vi "Set Channel by Name.vi"(8 "error in":errorcluster, 9 "Target":dbl, 10 "Channel Name":string, 11 "PRM in":refnum<class "PRM.lvclass">) -> (0 "error out":errorcluster, 3 "PRM out":refnum<class "PRM.lvclass">)   [LabVIEW 2019, in "PRM.lvlib" / "PRM.lvclass"]
uses:
  Library/PRM.lvclass
  C:/Users/Public/Documents/Development/builds/Instruments/Instruments.lvlibp/Library/Instruments.lvclass
  Library/PRM.lvclass/PRM.ctl
  Accessors/Write Active Channel.vi
  Accessors/Write Setting.vi
  Accessors/Read Active Channel.vi
  Accessors/Read Units.vi
  builds/Instruments/Instruments.lvlibp/Private/Polymorphic/Special/Event from String.vi
  builds/Instruments/Instruments.lvlibp/Accessors/Command with Logging.vi
  builds/Engine/Engine.lvlibp/Project/Engine.lvclass
  builds/Instruments/Instruments.lvlibp/Library/Instruments.lvclass
  builds/Instruments/Instruments.lvlibp
  C:/Users/Public/Documents/Development/builds/Engine/Engine.lvlibp/Project/Engine.lvclass
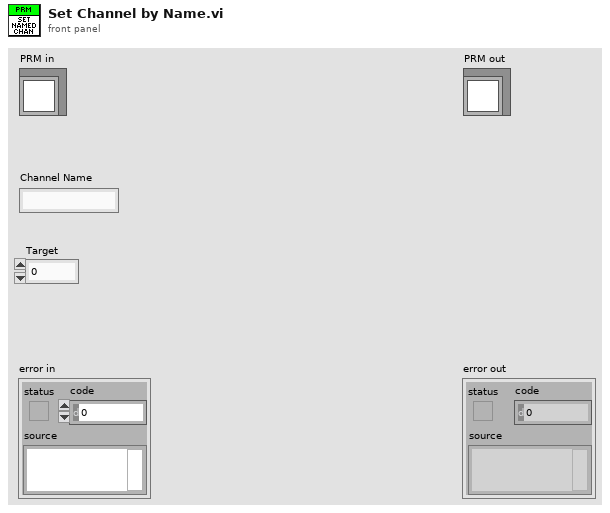
[diagram p1: front panel]
types:
  T1 = typedef "PRM.lvlib/PRM.lvclass/Units.ctl" = enum16{"Celsius", "Fahrenheit", "Kelvin", "Ohms"}
  T2 = cluster{"Timestamp":timestamp, "Description":string, "Data":string}
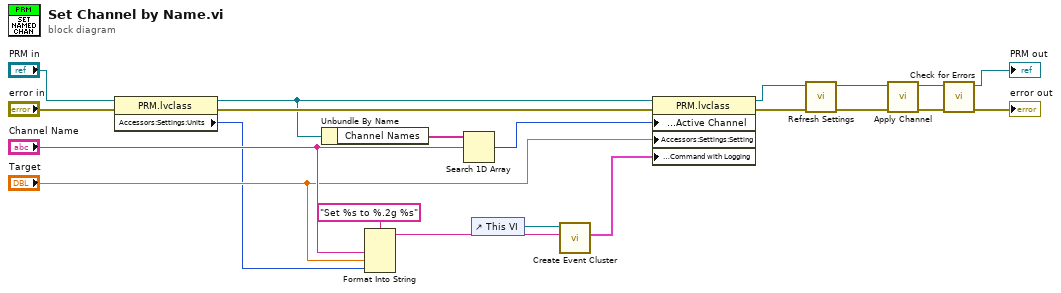
[diagram p0: block diagram]
diagram:
  n1 = property class="PRM.lvclass"(reference="PRM in", error in="error in") -> (reference out=w5:refnum<class "PRM.lvclass">, error out=w7:errorcluster, "Accessors:Settings:Units"=w4:T1)
  n2 = Unbundle By Name(w5) -> ("Channel Names"=w21:string[])
  n3 = Format Into String(format string="Set %s to %.2g %s", "Channel Name", "Target", w4) -> (resulting string=w8:string)  [unwired: 2 in, 1 out]
  n4 = Search 1D Array(1D array=w21, element="Channel Name") -> (index of element=w20:i32)  [unwired: 1 in]
  n5 = control-ref of="This VI"() -> (w12:refnum<vi>)
  n6 = call-poly "Create Event Cluster.vi"("Value"=w8, "VI Refnum"=w12) -> ("Event Data"=w13:T2)  [unwired: 9 in]
  n7 = property class="PRM.lvclass"(reference=w5, error in=w7, "Accessors:Settings:Active Channel"=w20, "Accessors:Settings:Setting"="Target", "Accessors:Logging:Command with Logging"=w13) -> (reference out=w2:refnum<class "PRM.lvclass">, error out=w18:errorcluster)
  n8 = call "Refresh Settings.vi"("error in"=w18, "PRM in"=w2) -> ("error out"=w3:errorcluster, "PRM out"=w1:refnum<class "PRM.lvclass">)  [unwired: 8 in]
  n9 = call-dynamic "Apply Channel.vi"("error in (no error)"=w3, "PRM in"=w1) -> ("error out"=w17:errorcluster, "PRM out"=w15:refnum<class "PRM.lvclass">)  [unwired: 8 in]
  n10 = call "Check for Errors.vi"("error in"=w17, "Engine in"=w15) -> ("error out"=→"error out":errorcluster, "Engine out"=→"PRM out":refnum<class "PRM.lvclass">)  [unwired: 8 in]
